vi "PusherServo Open.vi"(8 "PWMDeadband (ms)":T1={"Name"="Servo", "maxPositivePwm"=2.27, "minPositivePwm"=1.513, "centerPwm"=1.507, "maxNegativePwm"=1.5, "minNegativePwm"=0.743}, 11 "PWM Channel":T3) -> (0 "Error Out":errorcluster, 3 "ServoDeviceRef Out":T2)   [LabVIEW 2023, in "Feeder_ACT.lvlib"]
uses:
  Feeder_ACT.lvlib
  <vilib>/Rock Robotics/SystemInterfaces/DIO/FPGA_DIOPWMChannel.ctl
  <vilib>/Rock Robotics/WPI/PWM/Servo/WPI_ServoDeviceRef.ctl
  <vilib>/Rock Robotics/WPI/PWM/WPI_PWMDeadband.ctl
  <vilib>/Rock Robotics/WPI/PWM/WPI_PWMDeadband_ms.ctl
  <vilib>/Rock Robotics/WPI/PWM/WPI_PWMChannelCacheOp.ctl
  <vilib>/Rock Robotics/WPI/PWM/WPI_PWMPeriodMultiplier.ctl
  <vilib>/Rock Robotics/SystemInterfaces/NetworkCommunication/NetComm_UsageReport_ResourceType.ctl
panel:
  # "The HS-785HB sail winch servo with it's large drum wheel has 3 1/2 revolutions of travel for hauling in even the largest of sails. \nWith its dual ball bearing supported output shaft the HS-785HB will provide years of reliable service."
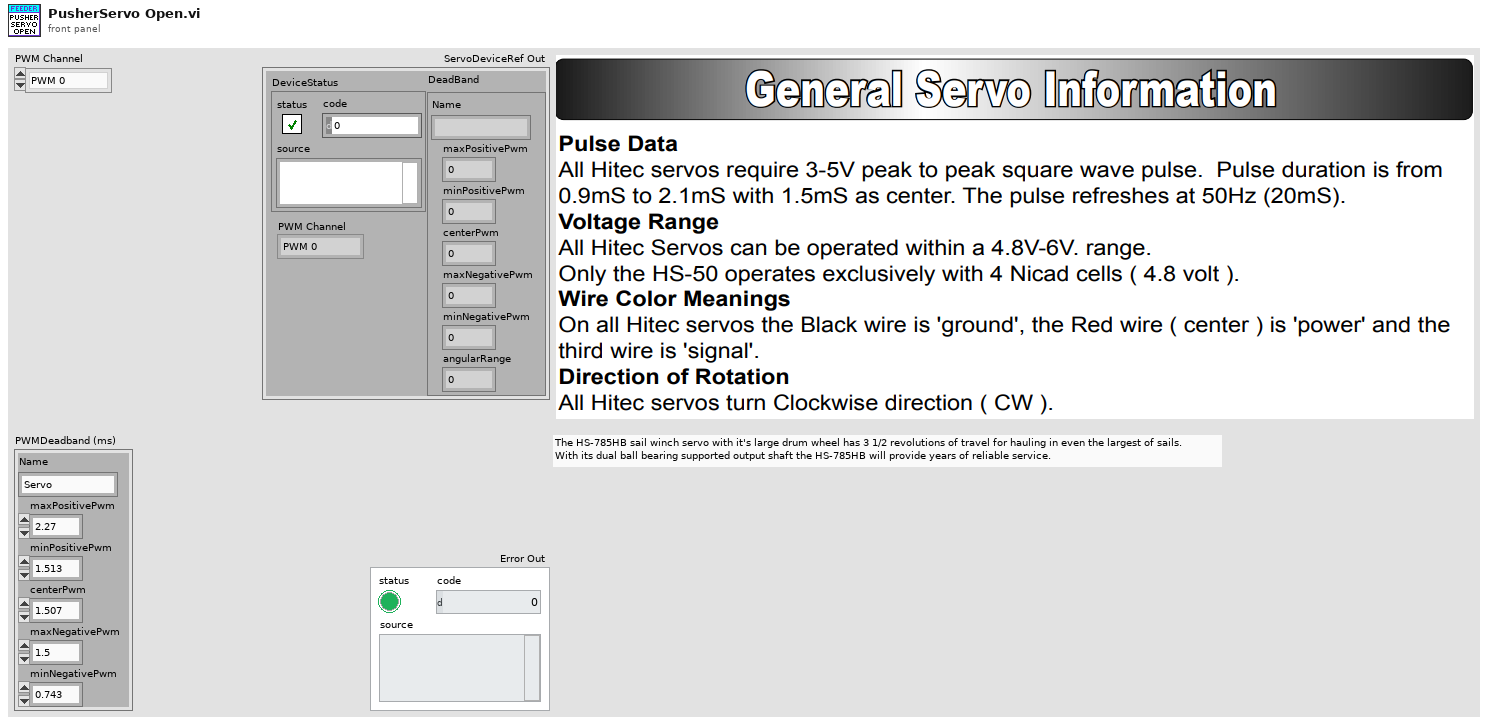
[diagram p1: front panel]
types:
  T1 = typedef "WPI_PWMDeadband_ms.ctl" = cluster{"Name":string, "maxPositivePwm":dbl, "minPositivePwm":dbl, "centerPwm":dbl, "maxNegativePwm":dbl, "minNegativePwm":dbl}
  T2 = typedef "WPI_ServoDeviceRef.ctl" = cluster{"DeviceStatus":errorcluster, "PWM Channel":T3, "DeadBand":T4}
  T3 = typedef "FPGA_DIOPWMChannel.ctl" = enum8{"PWM 0", "PWM 1", "PWM 2", "PWM 3", "PWM 4", "PWM 5", "PWM 6", "PWM 7", "PWM 8", "PWM 9", "PWM MXP 0", "PWM MXP 1", "PWM MXP 2", "PWM MXP 3", "PWM MXP 4", "PWM MXP 5", "PWM MXP 6", "PWM MXP 7", "PWM MXP 8", "PWM MXP 9", "Invalid"}
  T4 = typedef "WPI_PWMDeadband.ctl" = cluster{"Name":string, "maxPositivePwm":i32, "minPositivePwm":i32, "centerPwm":i32, "maxNegativePwm":i32, "minNegativePwm":i32, "angularRange":u16}
  T5 = typedef "NetComm_UsageReport_ResourceType.ctl" = enum8{"Controller", "Module", "Language", "CANPlugin", "Accelerometer", "ADXL345", "AnalogChannel", "AnalogTrigger", "AnalogTriggerOutput", "CANJaguar", "Compressor", "Counter", "Dashboard", "DigitalInput", "DigitalOutput", "DriverStationCIO", "DriverStationEIO", "DriverStationLCD", "Encoder", "GearTooth", "Gyro", "I2C", "Framework", "Jaguar", "Joystick", "Kinect", "KinectStick", "PIDController", "Preferences", "PWM", "Relay", "RobotDrive", "SerialPort", "Servo", "Solenoid", "SPI", "Task", "Ultrasonic", "Victor", "Button", "Command", "AxisCamera", "PCVideoServer", "SmartDashboard", "Talon", "HiTechnicColorSensor", "HiTechnicAccel", "HiTechnicCompass", "SRF08", "AnalogOutput", "Victor SP", "Talon SRX", "CAN Talon SRX", "ADXL362 Accel", "ADXRS450 Gyro", "Rev SPARK", "Mindsensors SD540", "Digital Filter", "ADIS16448", "PDP", "PCM", "PigeonIMU", "Nidec Brushless", "CTRE CANifier", "CTRE TalonFX", "CTRE Future 1", "CTRE Future 2", "CTRE Future 3", "CTRE Future 4", "CTRE Future 5", "CTRE Future 6", "Linear Filter", "Xbox Controller", "USB Camera", "NavX", "Pixy", "Pixy2", "ScanseSweep", "Shuffleboard", "CAN", "Digilent DMC60", "PWM Victor SPX", "Rev SPARK MAX PWM", "Rev SPARK MAX CAN", "ADIS16470", "PIDController2", "ProfiledPIDController", "Kinematics", "Odometry", "Units", "Trapezoid Profile", "DutyCycle", "Addressable LEDs", "Fusion Venom", "CTRE Future 7", "CTRE Future 8", "CTRE Future 9", "CTRE Future 10", "CTRE Future 11", "CTRE Future 12", "CTRE Future 13", "CTRE Future 14", "Exponential Profile", "PS4 Controller", "Photon Camera", "Photon Pose Estimator", "Path Planner Path", "Path Planner Auto", "Path Finding Command", "Redux Future 1", "Redux Future 2", "Redux Future 3", "Redux Future 4", "Redux Future 5", "Rev SPARK Flex CAN", "Rev SPARK Flex PWM"}
  T6 = typedef "WPI_PWMPeriodMultiplier.ctl" = u8
  T7 = typedef "WPI_PWMChannelCacheOp.ctl" = enum16{"Acquire", "Release", "Status"}
  T8 = typedef "WPI_PWMDeviceRef.ctl" = cluster{"DeviceStatus":errorcluster, "PWM Channel":T3}
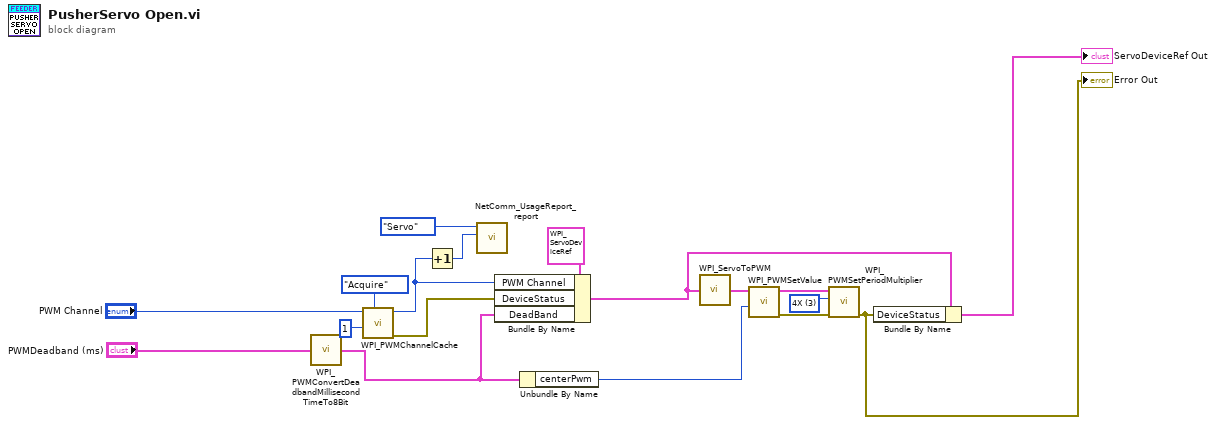
[diagram p0: block diagram]
diagram:
  w13 = T6 3 items=["1X"=0, "2X"=1, "4X"=3] ("PWMPeriodMultiplier")
  n1 = call <vilib>:"WPI_PWMConvertDeadbandMillisecondTimeTo8Bit.vi"("PWMDeadband (ms)"="PWMDeadband (ms)") -> ("PWMDeadband Coefficient"=w18:T4)  [unwired: 14 in]
  n2 = call <vilib>:"WPI_PWMChannelCache.vi"("Operation"=WPI_PWMChannelCacheOp."Acquire", "Additional Depth"=1, "PWMChannel"="PWM Channel") -> ("error out"=w7:errorcluster, "AllocatedPWMChannel"=w17:T3)  [unwired: 2 in, 5 out]
  n3 = Increment(x=w17) -> (x+1=w15:T3)
  n4 = call <vilib>:"NetComm_UsageReport_report.vi"("Instance Number"=w15, "Resource Type"=NetComm_UsageReport_ResourceType."Servo") -> ()  [unwired: 10 in]
  n5 = Bundle By Name(cluster=T2 {"DeviceStatus"={"status"=FALSE, "code"=0, "source"=""}, "PWM Channel"=enum."PWM 0", "DeadBand"={"Name"="", "maxPositivePwm"=0, "minPositivePwm"=0, "centerPwm"=0, "maxNegativePwm"=0, "minNegativePwm"=0, "angularRange"=0}} ("ServoDeviceRef in"), "PWM Channel"=w17, "DeviceStatus"=w7, "DeadBand"=w18) -> (w10:T2)
  n6 = Unbundle By Name(w18) -> ("centerPwm"=w8:i32)
  n7 = call <vilib>:"WPI_ServoToPWM.vi"("ServoDeviceRef"=w10) -> ("PWMDeviceRef"=w9:T8)
  n8 = call <vilib>:"WPI_PWMSetValue.vi"("Value"=w8, "PWMDeviceRef"=w9) -> ("error out"=w14:errorcluster, "PWMDeviceRef"=w12:T8)  [unwired: 2 in, 6 out]
  n9 = call <vilib>:"WPI_PWMSetPeriodMultiplier.vi"("error in (no error)"=w14, "PWMPeriodMultiplier"=w13, "PWMDeviceRef"=w12) -> ("error out"=w5:errorcluster)  [unwired: 8 out]
  "Error Out" <- w5
  n10 = Bundle By Name(cluster=w10, "DeviceStatus"=w5) -> (→"ServoDeviceRef Out":T2)
